vi "BooleanMeasure.vi"(5 "EndTime":timestamp, 7 "StartTime":timestamp, 8 "error in":errorcluster, 11 "BooleanMeasure":refnum<class "BooleanMeasure.lvclass">) -> (0 "error out":errorcluster, 3 "Passed":bool)   [LabVIEW 2020]
uses:
  ProligentResultProcessor/Measure/BooleanMeasure/BooleanMeasure.lvclass
  ProligentResultProcessor/Measure/BooleanMeasureLimit/BooleanMeasureLimit.lvclass
  ProligentResultProcessor/Measure/MeasureLimit/MeasureLimit.lvclass
  ProligentResultProcessor/Model/CustomData/CustomData.lvclass
  ProligentResultProcessor/Measure/Measure/Measure.lvclass
  C:/Projects/Result Processor/src/LabVIEWResultProcessor/ProligentResultProcessor/Measure/Measure/Measure.lvclass
  C:/Projects/Result Processor/src/LabVIEWResultProcessor/ProligentResultProcessor/Measure/BooleanMeasure/BooleanMeasure.lvclass
  C:/Projects/Result Processor/src/LabVIEWResultProcessor/ProligentResultProcessor/Measure/MeasureLimit/MeasureLimit.lvclass
  C:/Projects/Result Processor/src/LabVIEWResultProcessor/ProligentResultProcessor/Measure/BooleanMeasureLimit/BooleanMeasureLimit.lvclass
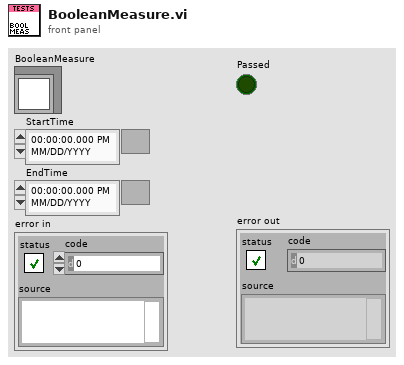
[diagram p1: front panel]
types:
  T1 = enum16{"PASS", "FAIL", "NOT_COMPLETED", "ABORTED"}
  T2 = typedef "ProligentResultProcessor.lvlib/ExecutionStatus.lvclass/Value.ctl" = enum16{"PASS", "FAIL", "NOT_COMPLETED", "ABORTED"}
  T3 = typedef "ProligentResultProcessor.lvlib/Measure.lvclass/Unit.ctl" = cluster{"Name":string, "Symbol":string}
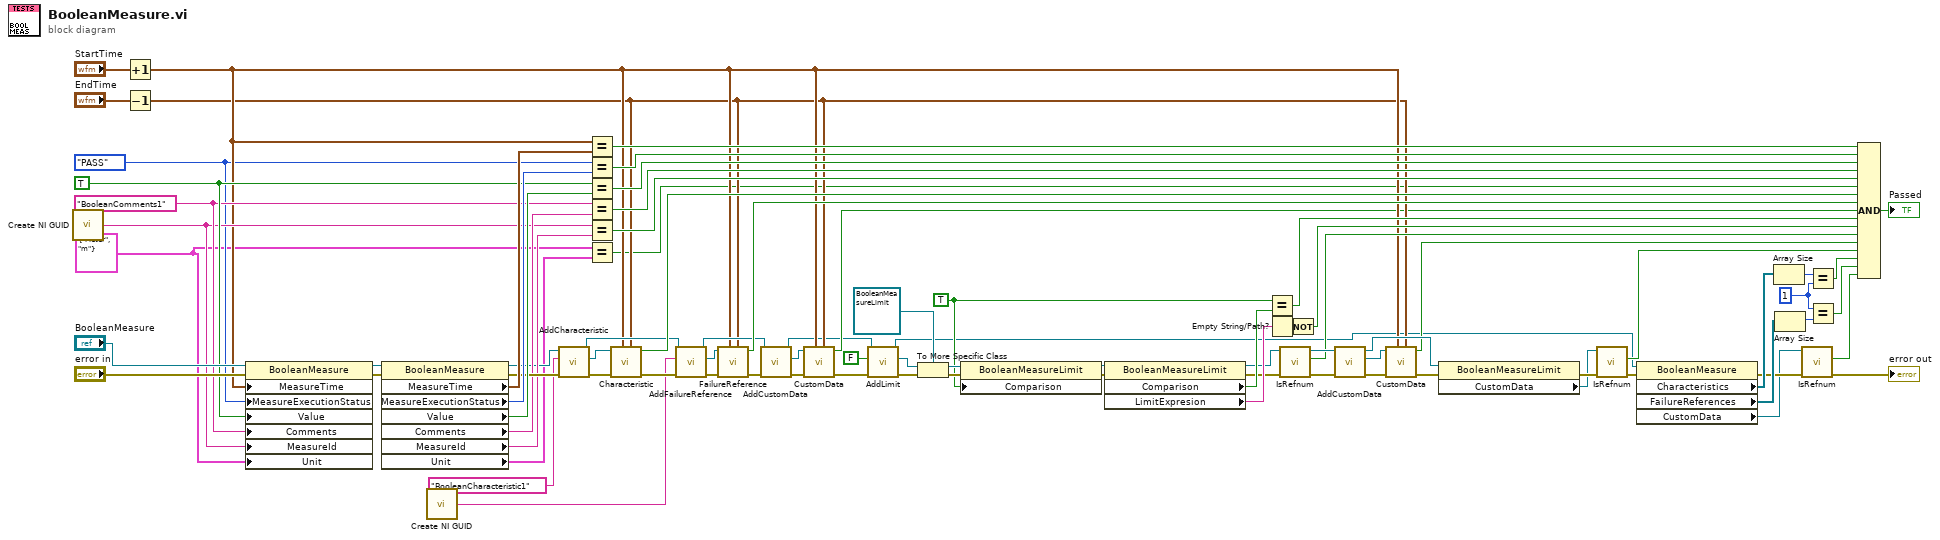
[diagram p0: block diagram]
diagram:
  w3 = cluster{"Name":string, "Symbol":string} {"Name"="Meter", "Symbol"="m"} ("Unit")
  w10 = 1 ("y")
  w45 = "BooleanComments1"
  w65 = TRUE ("Comparison")
  w73 = TRUE
  w19 = T1."PASS" ("ProcessRunStatus")
  n1 = call <vilib>:"Create NI GUID.vi"() -> ("NI GUID"=w43:string)
  n2 = Increment(x="StartTime") -> (x+1=w23:timestamp)
  n3 = Decrement(x="EndTime") -> (x-1=w22:timestamp)
  n4 = property class="BooleanMeasure"(reference="BooleanMeasure", error in="error in", "MeasureTime"=w23, "MeasureExecutionStatus"=w19, "Value"=w73, "Comments"=w45, "MeasureId"=w43, "Unit"=w3) -> (reference out=w83:refnum<class "BooleanMeasure.lvclass">, error out=w82:errorcluster)
  n5 = property class="BooleanMeasure"(reference=w83, error in=w82) -> (reference out=w36:refnum<class "BooleanMeasure.lvclass">, error out=w72:errorcluster, "MeasureTime"=w81:timestamp, "MeasureExecutionStatus"=w80:T2, "Value"=w79:bool, "Comments"=w44:string, "MeasureId"=w42:string, "Unit"=w2:T3)
  n6 = call <vilib>:"Create NI GUID.vi"() -> ("NI GUID"=w30:string)
  n7 = call "AddCharacteristic.vi"("error in (no error)"=w72, "FullName"="BooleanCharacteristic1", "Measure in"=w36) -> ("error out"=w37:errorcluster, "Characteristic"=w34:refnum<class "Characteristic.lvclass">, "Measure out"=w31:refnum<class "BooleanMeasure.lvclass">)  [unwired: 6 in]
  n8 = Equal?(x=w23, y=w81) -> (x = y?=w78:bool)
  n9 = Equal?(x=w19, y=w80) -> (x = y?=w46:bool)
  n10 = Equal?(x=w73, y=w79) -> (x = y?=w77:bool)
  n11 = Equal?(x=w45, y=w44) -> (x = y?=w41:bool)
  n12 = Equal?(x=w43, y=w42) -> (x = y?=w40:bool)
  n13 = Equal?(x=w3, y=w2) -> (x = y?=w1:bool)
  n14 = call "Characteristic.vi"("EndTime"=w22, "StartTime"=w23, "error in (no error)"=w37, "Characteristic in"=w34) -> ("error out"=w32:errorcluster, "Passed"=w33:bool)  [unwired: 6 in]
  n15 = call "AddFailureReference.vi"("error in (no error)"=w32, "Id"=w30, "Measure in"=w31) -> ("error out"=w18:errorcluster, "FailureReference"=w17:refnum<class "FailureReference.lvclass">, "Measure out"=w25:refnum<class "BooleanMeasure.lvclass">)  [unwired: 6 in]
  n16 = call "FailureReference.vi"("EndTime"=w22, "StartTime"=w23, "error in"=w18, "Defect"=w17) -> ("error out"=w29:errorcluster, "Passed"=w28:bool)  [unwired: 6 in]
  n17 = call "AddCustomData.vi"("error in (no error)"=w29, "Measure in"=w25) -> ("error out"=w26:errorcluster, "CustomData"=w24:refnum<class "CustomData.lvclass">, "Measure out"=w20:refnum<class "BooleanMeasure.lvclass">)  [unwired: 7 in]
  n18 = call "CustomData.vi"("EndTime"=w22, "StartTime"=w23, "error in"=w26, "CustomData"=w24) -> ("error out"=w27:errorcluster, "Passed"=w21:bool)  [unwired: 6 in]
  n19 = call "AddLimit.vi"("error in"=w27, "Comparison"=FALSE, "BooleanMeasure in"=w20) -> ("error out"=w38:errorcluster, "BooleanMeasureLimit"=w39:refnum<class "BooleanMeasureLimit.lvclass">, "BooleanMeasure out"=w15:refnum<class "BooleanMeasure.lvclass">)  [unwired: 6 in]
  n20 = To More Specific Class(target class=refnum<class "BooleanMeasureLimit.lvclass"> refnum ("ProligentResultProcessor:BooleanMeasureLimit"), reference=w39, error in=w38) -> (specific class reference=w68:refnum<class "BooleanMeasureLimit.lvclass">, error out=w70:errorcluster)
  n21 = property class="BooleanMeasureLimit"(reference=w68, error in=w70, "Comparison"=w65) -> (reference out=w67:refnum<class "BooleanMeasureLimit.lvclass">, error out=w66:errorcluster)
  n22 = property class="BooleanMeasureLimit"(reference=w67, error in=w66) -> (reference out=w55:refnum<class "BooleanMeasureLimit.lvclass">, error out=w60:errorcluster, "Comparison"=w64:bool, "LimitExpresion"=w63:string)
  n23 = Equal?(x=w65, y=w64) -> (x = y?=w62:bool)
  n24 = Empty String/Path?(string/path=w63) -> (empty?=w61:bool)
  n25 = call "IsRefnum.vi"("error in"=w60, "MeasureLimit in"=w55) -> ("error out"=w56:errorcluster, "IsRefnum"=w53:bool, "MeasureLimit out"=w54:refnum<class "BooleanMeasureLimit.lvclass">)  [unwired: 7 in]
  n26 = Not(x=w61) -> (.not. x?=w47:bool)
  n27 = call "AddCustomData.vi"("error in"=w56, "MeasureLimit in"=w54) -> ("error out"=w51:errorcluster, "CustomData"=w49:refnum<class "CustomData.lvclass">, "MeasureLimit out"=w52:refnum<class "BooleanMeasureLimit.lvclass">)  [unwired: 7 in]
  n28 = call "CustomData.vi"("EndTime"=w22, "StartTime"=w23, "error in"=w51, "CustomData"=w49) -> ("error out"=w50:errorcluster, "Passed"=w48:bool)  [unwired: 6 in]
  n29 = property class="BooleanMeasureLimit"(reference=w52, error in=w50) -> (error out=w59:errorcluster, "CustomData"=w58:refnum<class "CustomData.lvclass">)  [unwired: 1 out]
  n30 = call "IsRefnum.vi"("error in"=w59, "CustomDataType in"=w58) -> ("error out"=w16:errorcluster, "IsRefnum"=w57:bool)  [unwired: 7 in, 1 out]
  n31 = property class="BooleanMeasure"(reference=w15, error in=w16) -> (error out=w7:errorcluster, "Characteristics"=w14:refnum<class "Characteristic.lvclass">[], "FailureReferences"=w12:refnum<class "FailureReference.lvclass">[], "CustomData"=w5:refnum<class "CustomData.lvclass">)  [unwired: 1 out]
  n32 = Array Size(array=w14) -> (size(s)=w13:i32)
  n33 = Array Size(array=w12) -> (size(s)=w11:i32)
  n34 = call "IsRefnum.vi"("error in"=w7, "CustomDataType in"=w5) -> ("error out"=→"error out":errorcluster, "IsRefnum"=w4:bool)  [unwired: 7 in, 1 out]
  n35 = Equal?(x=w13, y=w10) -> (x = y?=w9:bool)
  n36 = Equal?(x=w10, y=w11) -> (x = y?=w8:bool)
  n37 = Compound Arithmetic op=AND(w78, w46, w77, w41, w40, w1, w33, w28, w21, w62, w47, w53, w48, w57, w9, w8, w4) -> (→"Passed":bool)
